vi "Y_H_change_data.vi"(8 "error in (no error)":errorcluster, 10 "SP_Set":dbl, 11 "Y_H_in":refnum<class "Y_H.lvclass">) -> (0 "error out":errorcluster, 3 "Y_H_out":refnum<class "Y_H.lvclass">)   [LabVIEW 2019, in "Y_H.lvclass"]
uses:
  Y_H.lvclass
  Y_H.lvclass/Y_H.ctl
  ctl/Y_H_state.ctl
  Timer Delay/Timers.lvlib
panel:
  in  "setpoint":T1(slide) caption="oC" scale=0.0..500.0 scale format="%#_5g"
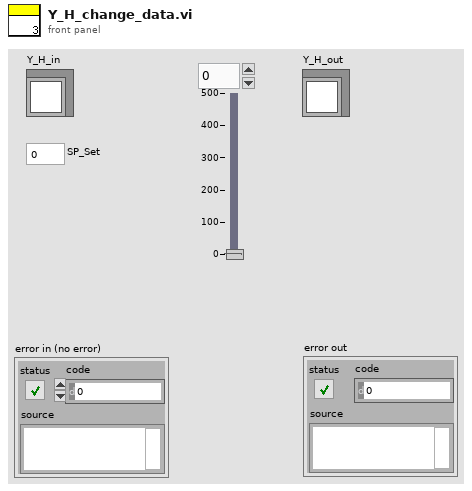
[diagram p1: front panel]
types:
  T1 = cluster{"Numeric":dbl, "Numeric":dbl, "Numeric":dbl}
  T2 = typedef "control.lvlib/Y_source.ctl" = enum8{"initialize", "local disabled", "local hand", "hand", "auto", "dist"}
  T3 = typedef "Y_H.lvclass/Y_H_state.ctl" = enum16{"init", "value change", "value not changed"}
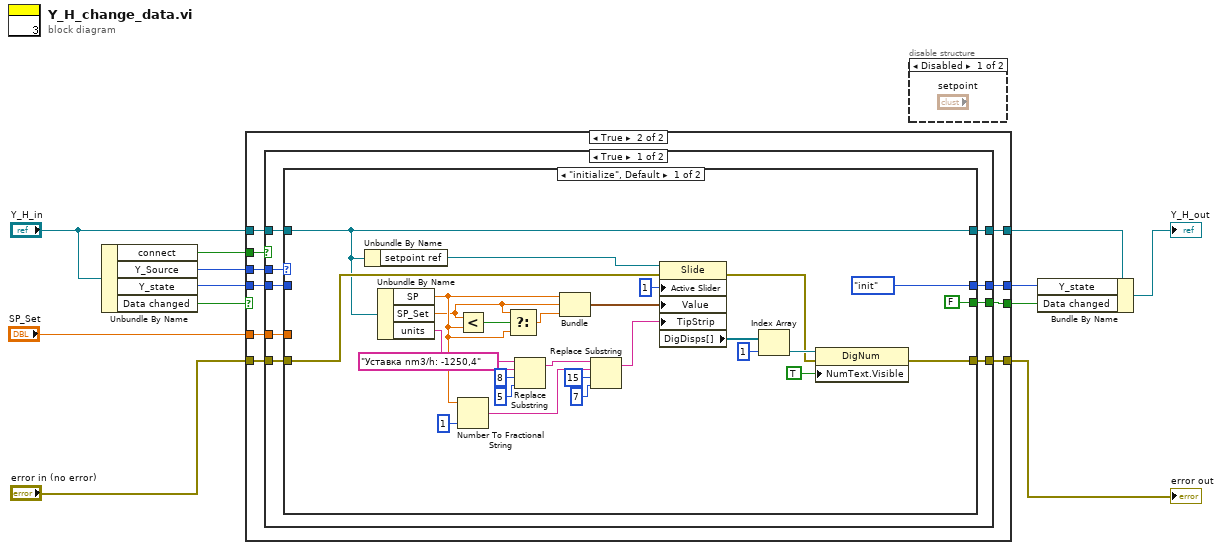
[diagram p0: block diagram]
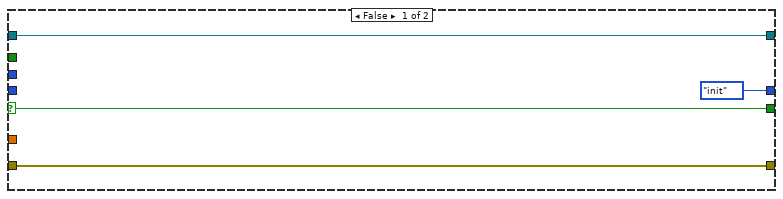
[diagram p2: hidden frame]
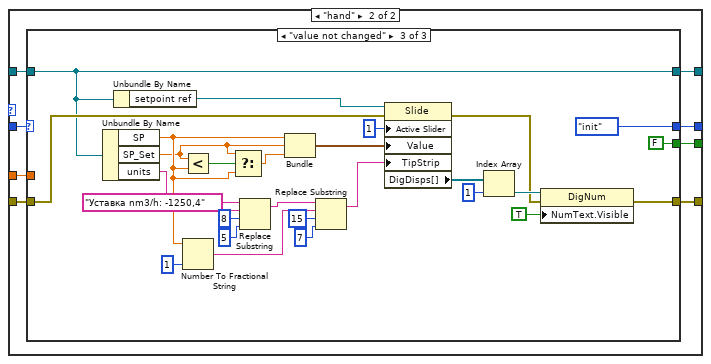
[diagram p3: hidden frame]
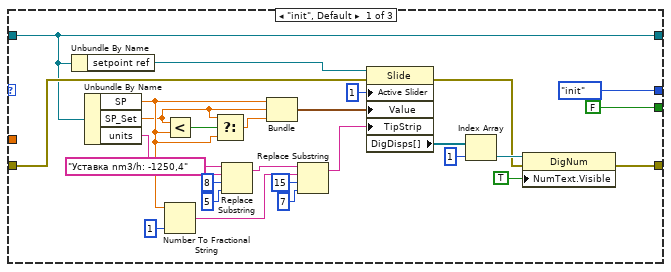
[diagram p4: hidden frame]
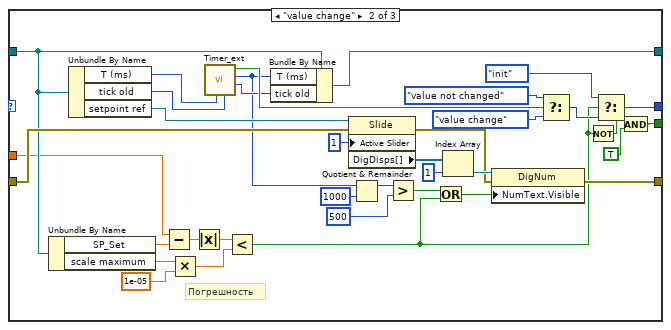
[diagram p5: hidden frame]
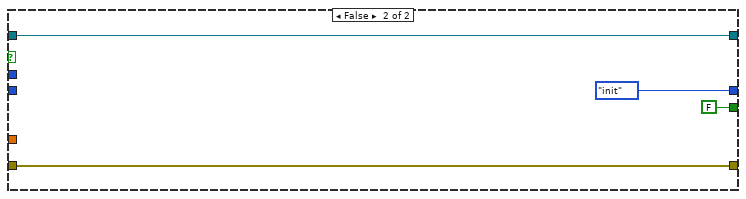
[diagram p6: hidden frame]
diagram:
  n1 = Unbundle By Name("Y_H_in") -> ("connect"=w8:bool, "Y_Source"=w7:T2, "Y_state"=w6:T3, "Data changed"=w2:bool)
  n2 = case shown="True" w2 {
    selector: w2 -> [w15 _]
    tunnel: [Y_H_state."init" ("switch_state") w26] -> w3
    tunnel: "error in (no error)" -> [w16 w25]
    tunnel: [w16 w24] -> w10
    tunnel: [w14 w23] -> w4
    tunnel: w8 -> [_ w22]
    tunnel: "Y_H_in" -> [w14 w21]
    tunnel: w7 -> [_ w20]
    tunnel: w6 -> [_ w19]
    tunnel: [w15 w18] -> w5
    tunnel: "SP_Set" -> [_ w17]
    frame False {
    }
    frame True {
      n3 = case shown="True" w22 {
        tunnel: w20 -> [w35 _]
        tunnel: [w32 w164] -> w23
        tunnel: [w34 Y_H_state."init" ("switch_state")] -> w26
        tunnel: w25 -> [w31 w162]
        tunnel: w21 -> [w33 w164]
        tunnel: [w30 w162] -> w24
        tunnel: w19 -> [w29 _]
        tunnel: [w28 FALSE] -> w18
        tunnel: w17 -> [w27 _]
        frame True {
          n4 = case shown="\"initialize\", Default" w35 {
            tunnel: [Y_H_state."init" ("switch_state") w69] -> w34
            tunnel: w33 -> [w53 w64]
            tunnel: [w53 w65] -> w32
            tunnel: w31 -> [w61 w70]
            tunnel: [w36 w68] -> w30
            tunnel: w29 -> [_ w67]
            tunnel: [FALSE w66] -> w28
            tunnel: w27 -> [_ w63]
            frame "initialize", Default {
              # "local hand"
              n5 = Unbundle By Name(w53) -> ("setpoint ref"=w62:refnum<vi>)
              n6 = Unbundle By Name(w53) -> ("SP"=w52:dbl, "SP_Set"=w51:dbl, "units"=w45:string)
              n7 = Less?(x=w51, y=w52) -> (x < y?=w59:bool)
              n8 = Number To Fractional String(number=w52, precision (6)=i16 1) -> (F-format string=w46:string)  [unwired: 2 in]
              n9 = Select(t=w51, s=w59, f=w52) -> (s? t:f=w58:dbl)
              n10 = Replace Substring(2:5 ("length (len. of substring)"), 3:8 ("offset (0)"), 4:w45, 5:"Уставка nm3/h: -1250,4") -> (1:w47:string)  [unwired: 1 out]
              n11 = Bundle("SP"=w52, "SP_Set"=w51, "SP"=w58) -> (w50:cluster{"SP":dbl, "SP_Set":dbl, "SP":dbl})  [unwired: 1 in]
              n12 = Replace Substring(2:7 ("length (len. of substring)"), 3:15 ("offset (0)"), 4:w46, 5:w47) -> (1:w44:string)  [unwired: 1 out]
              n13 = property on="Property Node" class="Slide"(reference=w62, error in=w61, "Active Slider"=1, "Value"=w50, "TipStrip"=w44) -> (error out=w37:errorcluster, "DigDisps[]"=w38:refnum<vi>[])  [unwired: 1 out]
              n14 = Index Array(array=w38, index=1) -> (element=w41:refnum<vi>)
              n15 = property class="DigNum"(reference=w41, error in=w37, "NumText.Visible"=TRUE ("Visible")) -> (error out=w36:errorcluster)  [unwired: 1 out]
            }
            frame "hand" {
              # "local hand"
              n16 = case shown="\"value not changed\"" w67 {
                tunnel: w70 -> [w97 w123 w159]
                tunnel: w64 -> [w94 w114 w134]
                tunnel: [Y_H_state."init" ("switch_state") w102 Y_H_state."init" ("switch_state")] -> w69
                tunnel: [w71 w128 w137] -> w68
                tunnel: [FALSE w101 FALSE] -> w66
                tunnel: [w94 w116 w134] -> w65
                tunnel: w63 -> [_ w113 _]
                frame "init", Default {
                  n17 = Unbundle By Name(w94) -> ("setpoint ref"=w93:refnum<vi>)
                  n18 = Unbundle By Name(w94) -> ("SP"=w85:dbl, "SP_Set"=w84:dbl, "units"=w78:string)
                  n19 = Less?(x=w84, y=w85) -> (x < y?=w91:bool)
                  n20 = Number To Fractional String(number=w85, precision (6)=i16 1) -> (F-format string=w79:string)  [unwired: 2 in]
                  n21 = Select(t=w84, s=w91, f=w85) -> (s? t:f=w90:dbl)
                  n22 = Replace Substring(2:5 ("length (len. of substring)"), 3:8 ("offset (0)"), 4:w78, 5:"Уставка nm3/h: -1250,4") -> (1:w80:string)  [unwired: 1 out]
                  n23 = Bundle("SP"=w85, "SP_Set"=w84, "SP"=w90) -> (w83:cluster{"SP":dbl, "SP_Set":dbl, "SP":dbl})  [unwired: 1 in]
                  n24 = Replace Substring(2:7 ("length (len. of substring)"), 3:15 ("offset (0)"), 4:w79, 5:w80) -> (1:w77:string)  [unwired: 1 out]
                  n25 = property on="Property Node" class="Slide"(reference=w93, error in=w97, "Active Slider"=1, "Value"=w83, "TipStrip"=w77) -> (error out=w72:errorcluster, "DigDisps[]"=w73:refnum<vi>[])  [unwired: 1 out]
                  n26 = Index Array(array=w73, index=1) -> (element=w76:refnum<vi>)
                  n27 = property class="DigNum"(reference=w76, error in=w72, "NumText.Visible"=TRUE ("Visible")) -> (error out=w71:errorcluster)  [unwired: 1 out]
                }
                frame "value change" {
                  # "Погрешность"
                  n28 = Unbundle By Name(w114) -> ("SP_Set"=w112:dbl, "scale maximum"=w110:dbl)
                  n29 = Unbundle By Name(w114) -> ("T (ms)"=w122:u32, "tick old"=w121:u32, "setpoint ref"=w124:refnum<vi>)
                  n30 = Subtract(x=w113, y=w112) -> (x-y=w111:dbl)
                  n31 = Multiply(x=w110, y=1e-05) -> (x*y=w107:dbl)
                  n32 = Absolute Value(x=w111) -> (abs(x)=w108:dbl)
                  n33 = call "Timer_ext.vi"("tick old"=w121, "t ms old"=w122) -> ("tick"=w117:u32, "t ms"=w115:u32, "End"=w120:bool)  [unwired: 7 in]
                  n34 = Less?(x=w108, y=w107) -> (x < y?=w99:bool)
                  n35 = Bundle By Name(cluster=w114, "T (ms)"=w115, "tick old"=w117) -> (w116:refnum<class "Y_H.lvclass">)
                  n36 = property on="Property Node" class="Slide"(reference=w124, error in=w123, "Active Slider"=1) -> (error out=w129:errorcluster, "DigDisps[]"=w130:refnum<vi>[])  [unwired: 1 out]
                  n37 = Quotient & Remainder(x=w115, y=u32 1000) -> (x-y*floor(x/y)=w125:u32)  [unwired: 1 out]
                  n38 = Greater?(x=w125, y=u32 500) -> (0:w105:bool)
                  n39 = Or(x=w105, y=w99) -> (x .or. y?=w106:bool)
                  n40 = Index Array(array=w130, index=1) -> (element=w131:refnum<vi>)
                  n41 = property class="DigNum"(reference=w131, error in=w129, "NumText.Visible"=w106) -> (error out=w128:errorcluster)  [unwired: 1 out]
                  n42 = Select(t=Y_H_state."value not changed" ("switch_state"), s=w120, f=Y_H_state."value change" ("switch_state")) -> (s? t:f=w104:T3)
                  n43 = Not(x=w99) -> (.not. x?=w98:bool)
                  n44 = Select(t=Y_H_state."init" ("switch_state"), s=w99, f=w104) -> (s? t:f=w102:T3)
                  n45 = And(x=w98, y=TRUE) -> (x .and. y?=w101:bool)
                }
                frame "value not changed" {
                  n46 = Unbundle By Name(w134) -> ("SP"=w151:dbl, "SP_Set"=w150:dbl, "units"=w144:string)
                  n47 = Unbundle By Name(w134) -> ("setpoint ref"=w160:refnum<vi>)
                  n48 = Less?(x=w150, y=w151) -> (x < y?=w157:bool)
                  n49 = Number To Fractional String(number=w151, precision (6)=i16 1) -> (F-format string=w145:string)  [unwired: 2 in]
                  n50 = Select(t=w150, s=w157, f=w151) -> (s? t:f=w156:dbl)
                  n51 = Replace Substring(2:5 ("length (len. of substring)"), 3:8 ("offset (0)"), 4:w144, 5:"Уставка nm3/h: -1250,4") -> (1:w146:string)  [unwired: 1 out]
                  n52 = Bundle("SP"=w151, "SP_Set"=w150, "SP"=w156) -> (w149:cluster{"SP":dbl, "SP_Set":dbl, "SP":dbl})  [unwired: 1 in]
                  n53 = Replace Substring(2:7 ("length (len. of substring)"), 3:15 ("offset (0)"), 4:w145, 5:w146) -> (1:w143:string)  [unwired: 1 out]
                  n54 = property on="Property Node" class="Slide"(reference=w160, error in=w159, "Active Slider"=1, "Value"=w149, "TipStrip"=w143) -> (error out=w138:errorcluster, "DigDisps[]"=w139:refnum<vi>[])  [unwired: 1 out]
                  n55 = Index Array(array=w139, index=1) -> (element=w140:refnum<vi>)
                  n56 = property class="DigNum"(reference=w140, error in=w138, "NumText.Visible"=TRUE ("Visible")) -> (error out=w137:errorcluster)  [unwired: 1 out]
                }
              }
            }
          }
        }
        frame False {
        }
      }
    }
  }
  "error out" <- w10
  n57 = disable-structure shown="Disabled" {
    frame Disabled {
    }
    frame Enabled {
    }
  }
  n58 = Bundle By Name(cluster=w4, "Y_state"=w3, "Data changed"=w5) -> (→"Y_H_out":refnum<class "Y_H.lvclass">)
